vi "GetSetParameterGroup.vi"(7 "error in":errorcluster, 8 "Parameter group number (1-4)":u8=1 min=1 max=4 step=1, 9 "get/set":T1, 10 "VISA resource name":refnum<visa-resource-name>) -> (0 "error out":errorcluster, 2 "Parameter group response":string, 3 "VISA resource name out":refnum<visa-resource-name>)   [LabVIEW 2023, in "Thermotron 8800.lvlib"]
doc: "PRMG\nCommand name: Send or load parameter group\nCommand type: Variable; edit from hold\nDescription: Queries the 8800 for the number of the parameter group that it is currently using. If the 8800 is in manual mode, the operation command selects the parameter group (1 through 4) that the 8800 will use to control the channels. Edit from hold operations temporarily change the parameter group for the program.\nSyntax: PRMG? or PRMG[,]d\nWhere d is the parameter group number (1 through 4).\nData type: Integer; see Syntax.\nQuery example: PRMG?\n8800 response: 2 (The 8800 is currently using parameter group 2.)\nOperation example: PRMG3\n8800 response: 0 (In manual mode, the 8800 will use parameter group 3.)"
uses:
  Thermotron 8800.lvlib
  Private/get set.ctl
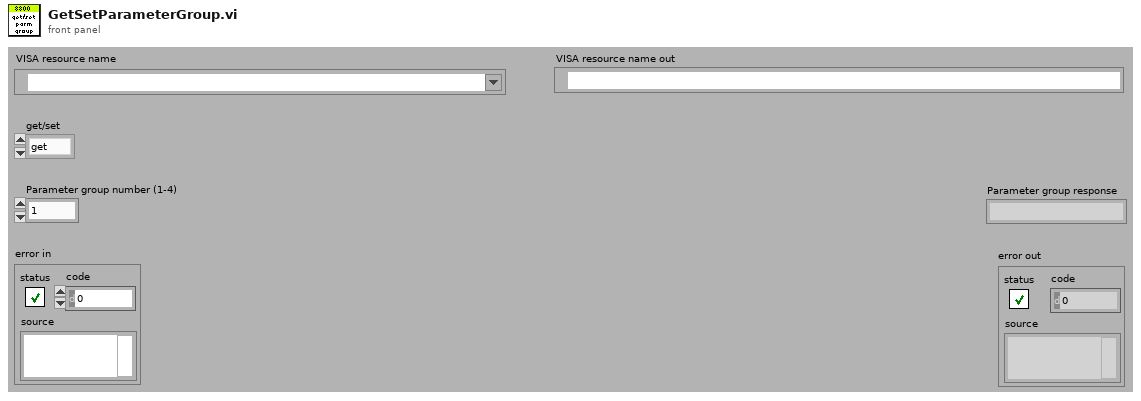
[diagram p1: front panel]
types:
  T1 = typedef "Thermotron 8800.lvlib/get set.ctl" = enum16{"get", "set"}
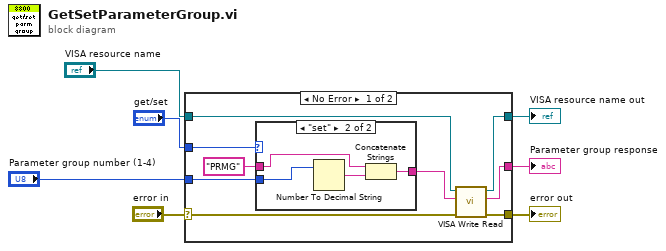
[diagram p0: block diagram]
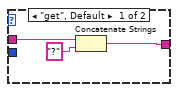
[diagram p2: hidden frame]
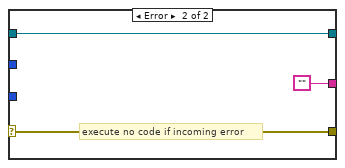
[diagram p3: hidden frame]
diagram:
  n1 = case shown="No Error" "error in" {
    selector: "error in" -> [w16 w25]
    tunnel: [w13 w26] -> w6
    tunnel: "VISA resource name" -> [w14 w26]
    tunnel: [w15 w25] -> w4
    tunnel: [w12 ""] -> w3
    tunnel: "get/set" -> [w11 _]
    tunnel: "Parameter group number (1-4)" -> [w9 _]
    frame No Error {
      n2 = case shown="\"set\"" w11 {
        tunnel: "PRMG" ("8800 Command") -> [w18 w21]
        tunnel: [w17 w20] -> w8
        tunnel: w9 -> [_ w23]
        frame "get", Default {
          n3 = Concatenate Strings(w18, "?" ("8800 Command")) -> (w17:string)
        }
        frame "set" {
          n4 = Number To Decimal String(number=w23) -> (decimal integer string=w22:string)  [unwired: 1 in]
          n5 = Concatenate Strings(w21, w22) -> (w20:string)
        }
      }
      n6 = call "VISA Write Read.vi"("error in (no error)"=w16, "8800 Command"=w8, "VISA Refnum in"=w14) -> ("error out"=w15:errorcluster, "read buffer"=w12:string, "VISA Refnum out"=w13:refnum<visa-resource-name>)  [unwired: 6 in]
    }
    frame Error {
      # "execute no code if incoming error"
    }
  }
  "VISA resource name out" <- w6
  "error out" <- w4
  "Parameter group response" <- w3
